vi "Do.vi"(8 "error in (no error)":errorcluster, 10 "Actor in":refnum<class "Simple Actor.lvclass">, 11 "Quit Msg in":refnum<class "Quit Msg.lvclass">) -> (0 "error out":errorcluster, 2 "Actor out":refnum<class "Simple Actor.lvclass">, 3 "Quit Msg out":refnum<class "Quit Msg.lvclass">)   [LabVIEW 2020, in "Simple Actor.lvlib" / "Quit Msg.lvclass"]
uses:
  Quit Msg.lvclass
  Simple Actor/Simple Actor.lvclass
  <vilib>/Utility/error.llb/Error Cluster From Error Code.vi
  <vilib>/ErrorRing/Error Ring.xnode
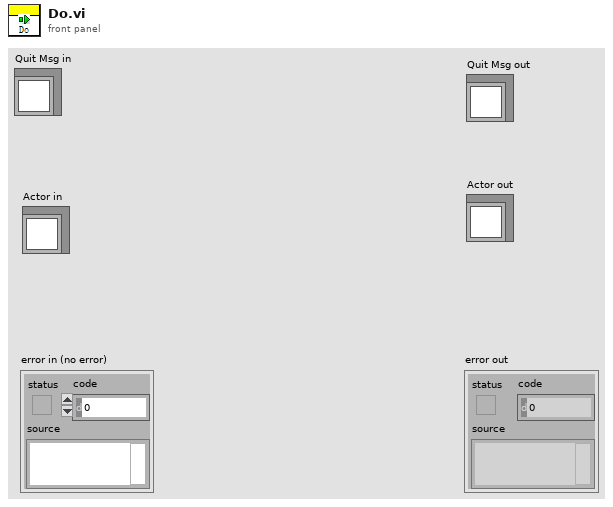
[diagram p1: front panel]
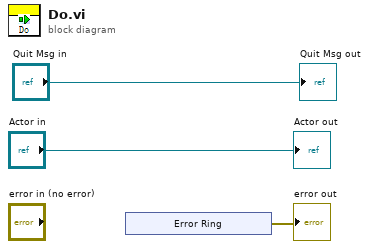
[diagram p0: block diagram]
diagram:
  n1 = xnode "Error Ring"() -> ("error out"=→"error out":errorcluster)
  "Actor out" <- "Actor in"
  "Quit Msg out" <- "Quit Msg in"
